vi "DT_Find Next Triangulation_Main.vi"(9 "Data In":T1, 10 "Triangles In":i32[][](array[numeric]), 11 "Points In":cluster{"x":dbl, "y":dbl, "index":i32}[](array[cluster])) -> (1 "Data Out":T1, 2 "Triangles Out":i32[][](array[numeric]), 3 "Points Out":cluster{"x":dbl, "y":dbl, "index":i32}[](array[cluster]))   [LabVIEW 2020, in "NI_AAL_Geometry.lvlib"]
uses:
  <vilib>/Analysis/NI_AAL_Geometry.lvlib
  <vilib>/Analysis/geometry.llb/DT_Find Next Triangulation_Data.ctl
  <vilib>/Analysis/geometry.llb/DT_Cal Length.vi
  <vilib>/Analysis/baseanly.llb/Determinant.vi
  <vilib>/Analysis/baseanly.llb/Real Determinant.vi
  <vilib>/Analysis/geometry.llb/DT_Triangle Manager_Get Adj_by Point.vi
  <vilib>/Analysis/geometry.llb/DT_Triangle Manager_Get Adj Ghost.vi
  <vilib>/Analysis/geometry.llb/DT_Triangle Manager_Get Adj Point_by Edge.vi
  <vilib>/Analysis/geometry.llb/DT_Triangle Manager_Format Ghost.vi
  <vilib>/Analysis/geometry.llb/DT_Triangle Manager_Get Oppo Point_in Ghost.vi
  <vilib>/Analysis/geometry.llb/DT_Triangle Manager_Get Oppo Point.vi
  <vilib>/Analysis/geometry.llb/DT_Triangle Manager_Default Ghost Index.vi
  <vilib>/Analysis/geometry.llb/DT_Triangle Manager_Get Ghost Point.vi
  <vilib>/Analysis/geometry.llb/DT_Triangle Manager_Get Oppo Edge.vi
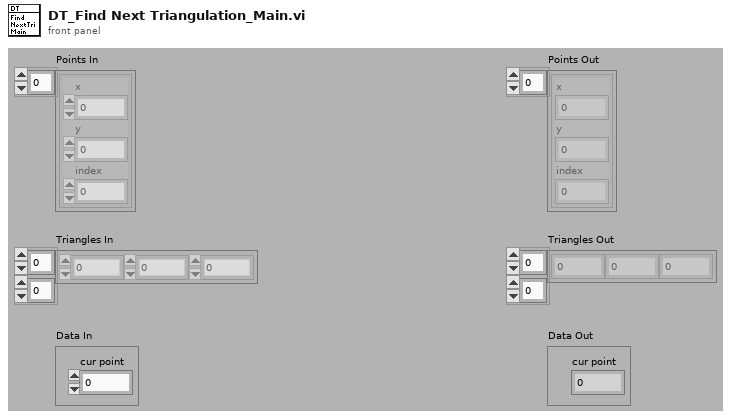
[diagram p1: front panel]
types:
  T1 = typedef "NI_AAL_Geometry.lvlib/DT_Find Next Triangulation_Data.ctl" = cluster{"cur point":i32, "cur triangle":i32, "cur local idx":i32, "base point":i32, "base triangle":i32, "base local idx":i32, "Candidate Triangles":i32[], "Candidate Point Idx":i32[]}
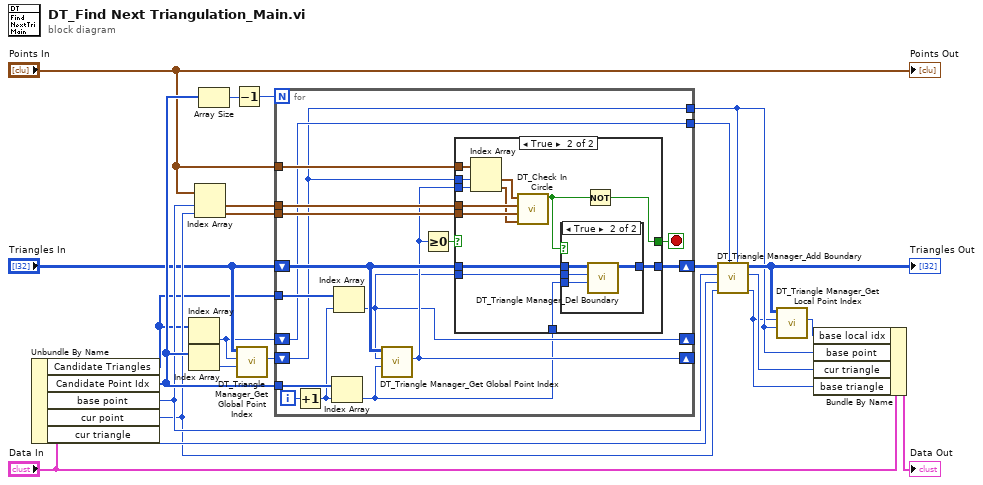
[diagram p0: block diagram]
diagram:
  n1 = Unbundle By Name("Data In") -> ("Candidate Triangles"=w6:i32[], "Candidate Point Idx"=w20:i32[], "base point"=w16:i32, "cur point"=w14:i32, "cur triangle"=w15:i32)
  n2 = Index Array(array=w6) -> (element=w3:i32)  [unwired: 1 in]
  n3 = Index Array(array=w20) -> (element=w7:i32)  [unwired: 1 in]
  n4 = Index Array(array="Points In", index #1=w16, index #2=w14) -> (element #1=w22:cluster{"x":dbl, "y":dbl, "index":i32}, element #2=w21:cluster{"x":dbl, "y":dbl, "index":i32})
  n5 = Array Size(array=w20) -> (size(s)=w23:i32)
  n6 = Decrement(x=w23) -> (x-1=w9:i32)
  n7 = call <vilib>:"DT_Triangle Manager_Get Global Point Index.vi"("local idx"=w7, "triangle"=w3, "Triangles"="Triangles In") -> ("global idx"=w8:i32)  [unwired: 8 out]
  n8 = for {
    N: w9 -> [_]
    tunnel: w20 -> [w38]
    tunnel: w22 -> [w36]
    tunnel: w21 -> [w35]
    shift-right: [w34] -> w17
    shift-left: "Triangles In" -> [w31]
    tunnel: w6 -> [w32]
    shift-right: [w28] -> _
    shift-left: w8 -> [w25]
    tunnel: [w26] -> w5
    tunnel: [w25] -> w4
    shift-right: [w27] -> _
    shift-left: w3 -> [w26]
    tunnel: "Points In" -> [w37]
    i -> [w39]
    stop <- w29 stop-if-true
    n9 = Increment(x=w39) -> (x+1=w33:i32)
    n10 = Index Array(array=w38, index=w33) -> (element=w24:i32)
    n11 = Index Array(array=w32, index=w33) -> (element=w27:i32)
    n12 = call <vilib>:"DT_Triangle Manager_Get Global Point Index.vi"("local idx"=w24, "triangle"=w27, "Triangles"=w31) -> ("global idx"=w28:i32)  [unwired: 8 out]
    n13 = Greater Or Equal To 0?(x=w28) -> (x >= 0?=w30:bool)
    n14 = case shown="True" w30 {
      selector: w30 -> [w41 _]
      tunnel: w37 -> [_ w54]
      tunnel: w36 -> [_ w52]
      tunnel: w35 -> [_ w51]
      tunnel: [w40 w49] -> w34
      tunnel: w28 -> [_ w48]
      tunnel: w25 -> [_ w47]
      tunnel: w31 -> [w40 w46]
      tunnel: w27 -> [_ w43]
      tunnel: [w41 w44] -> w29
      tunnel: w24 -> [_ w42]
      frame False {
      }
      frame True {
        n15 = Index Array(array=w54, index #1=w47, index #2=w48) -> (element #1=w53:cluster{"x":dbl, "y":dbl, "index":i32}, element #2=w50:cluster{"x":dbl, "y":dbl, "index":i32})
        n16 = call <vilib>:"DT_Check In Circle.vi"("p 4"=w50, "p 3"=w51, "p 2"=w52, "p 1"=w53) -> ("in circle?"=w45:bool)  [unwired: 7 out]
        n17 = case shown="True" w45 {
          tunnel: w46 -> [w55 w59]
          tunnel: [w55 w58] -> w49
          tunnel: w43 -> [_ w57]
          tunnel: w42 -> [_ w56]
          frame False {
          }
          frame True {
            n18 = call <vilib>:"DT_Triangle Manager_Del Boundary.vi"("point idx"=w56, "triangle in"=w57, "Triangles In"=w59) -> ("Triangles Out"=w58:i32[][])  [unwired: 8 out]
          }
        }
        n19 = Not(x=w45) -> (.not. x?=w44:bool)
      }
    }
  }
  n20 = call <vilib>:"DT_Triangle Manager_Add Boundary.vi"("point 2"=w4, "triangle 2"=w5, "point 1"=w14, "triangle 1"=w15, "apex point"=w16, "Triangles In"=w17) -> ("new triangle 2"=w2:i32, "triangle"=w13:i32, "Triangles Out"=w12:i32[][])  [unwired: 1 in, 2 out]
  "Triangles Out" <- w12
  n21 = call <vilib>:"DT_Triangle Manager_Get Local Point Index.vi"("global idx"=w4, "triangle"=w2, "Triangles"=w12) -> ("local idx"=w11:i32)  [unwired: 8 out]
  n22 = Bundle By Name(cluster="Data In", "base local idx"=w11, "base point"=w4, "cur triangle"=w13, "base triangle"=w2) -> (→"Data Out":T1)
  "Points Out" <- "Points In"
